vi "reset.vi"(8 "error in (no error)":errorcluster, 11 "DL090215DataCollection in":refnum<class "DataCollectionDL090215.lvclass">) -> (0 "error out":errorcluster, 3 "DL090215DataCollection out":refnum<class "DataCollectionDL090215.lvclass">)   [LabVIEW 2010, in "DataCollectionDL090215.lvclass"]
uses:
  DataCollectionDL090215.lvclass
  common/classes/ImageCollection/ImageCollection/ImageCollection.lvclass
  DataCollectionDL090215.lvclass/DataCollectionDL090215.ctl
  common/classes/ErrorController/ErrorController/class_data.vi
  common/classes/ErrorController/ErrorController/ErrorController.lvclass
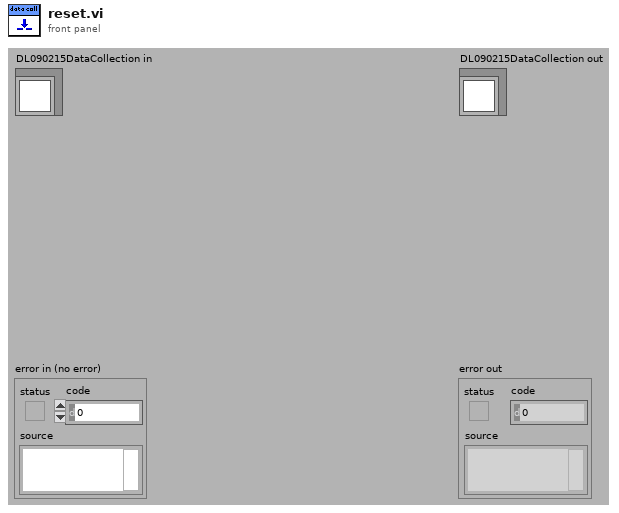
[diagram p1: front panel]
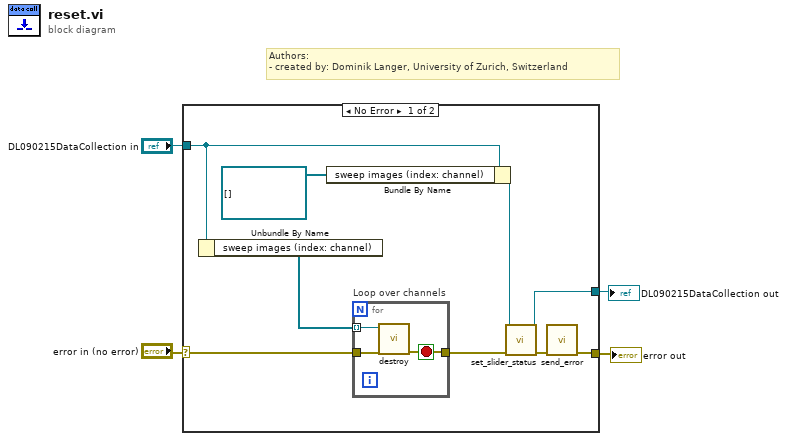
[diagram p0: block diagram]
diagram:
  # "Authors: \n- created by: Dominik Langer, University of Zurich, Switzerland"
  n1 = case shown="No Error" "error in (no error)" {
    selector: "error in (no error)" -> [w12 w18]
    tunnel: [w5 w18] -> w3
    tunnel: [w7 w17] -> w1
    tunnel: "DL090215DataCollection in" -> [w13 w17]
    frame No Error {
      n2 = Unbundle By Name(w13) -> ("sweep images (index: channel)"=w11:refnum<class "ImageCollection.lvclass">[])
      n3 = Bundle By Name(cluster=w13, "sweep images (index: channel)"=refnum<class "ImageCollection.lvclass">[] []) -> (w8:refnum<class "DataCollectionDL090215.lvclass">)
      n4 = for "Loop over channels" {
        tunnel: w11 -> [w15] mode=indexing
        tunnel: w12 -> [w16]
        tunnel: [w14] -> w9
        stop <- w14 stop-if-true
        n5 = call-dynamic "destroy.vi"("error in (no error)"=w16, "ImageCollection in"=w15) -> ("error out"=w14:errorcluster)  [unwired: 9 out]
      }
      n6 = call-dynamic "set_slider_status.vi"("error in (no error)"=w9, "DL090215DataCollection in"=w8) -> ("error out"=w6:errorcluster, "DL090215DataCollection out"=w7:refnum<class "DataCollectionDL090215.lvclass">)  [unwired: 8 out]
      n7 = call "send_error.vi"("error in (no error)"=w6) -> ("error out"=w5:errorcluster)  [unwired: 10 in]
    }
    frame Error {
    }
  }
  "error out" <- w3
  "DL090215DataCollection out" <- w1
